vi "Incomplete Elliptic Integral F.vi"(10 "a":dbl=1.5707963267948966 format="%.2f", 11 "k":dbl format="%.2f") -> (3 "F(k, a)":dbl format="%.2f")   [LabVIEW 2017, in "NI_Gmath.lvlib"]
doc: "Computes the Legendre elliptic integral of the first kind. You must manually select the polymorphic instance you want to use."
uses:
  NI_Gmath.lvlib
  lvanlys.dll
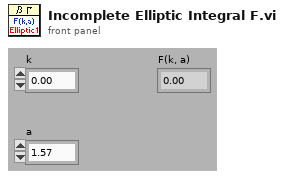
[diagram p1: front panel]
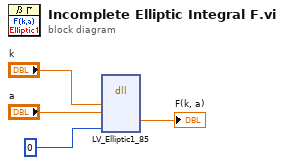
[diagram p0: block diagram]
diagram:
  n1 = dll-call lib="C:/Program Files/National Instruments/LabVIEW 2017/resource/lvanlys.*" fn="LV_Elliptic1_85"("k"="k", "a"="a", "funcType"=0) -> ("Elliptic1(k, a)"=→"F(k, a)":dbl)  [unwired: 8 in, 2 out]
